vi "Manual worksheet input.vi"() -> (0 "error out":errorcluster, 1 "data names":string[](array[string]), 2 "file numbers":string[](array[string]), 3 "Data clusters":cluster{"array type (2D Dbl)":dbl[][]}[](array[cluster]))   [LabVIEW 2019]
panel:
  in  "dataset name (option)":string="data"
  in  "OK":bool=TRUE
  out "XY Graph":T1(graph)
  in  "XY data worksheet":string
  # "Worksheet has a format below (2n colums)\nx1, y1, x2, y2, x3, y3,... xn, yn\n\nConvert to datasets of individual n XY plots such as  (x1, y1), (x2, y2), ...(xn,yn)."
  # "(Copy and Paste multiple XY data set)"
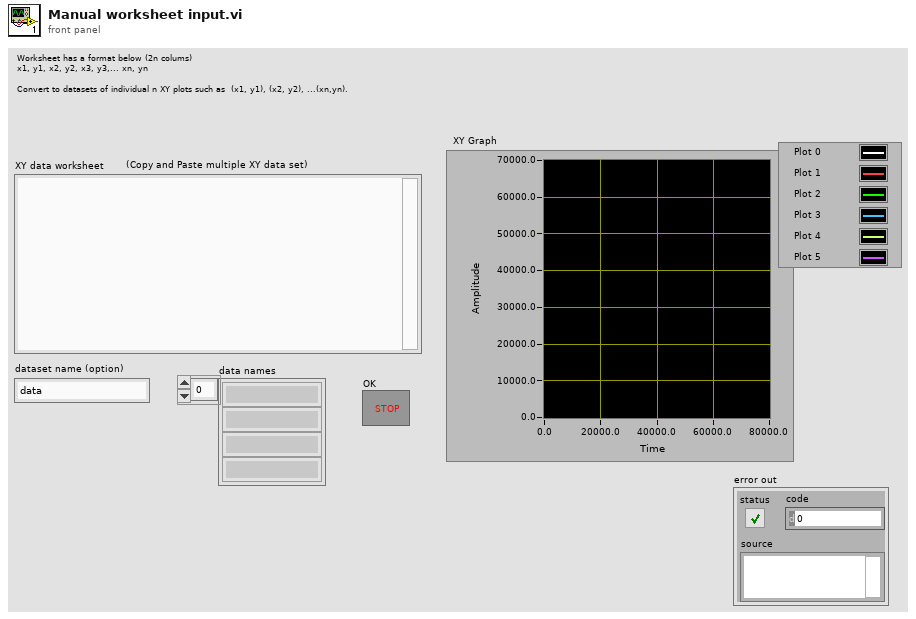
[diagram p1: front panel]
types:
  T1 = cluster{"array type (2D Dbl)":dbl[], "array type (2D Dbl)":dbl[]}[]
  T2 = cluster{"array type (2D Dbl)":dbl[], "array type (2D Dbl)":dbl[]}
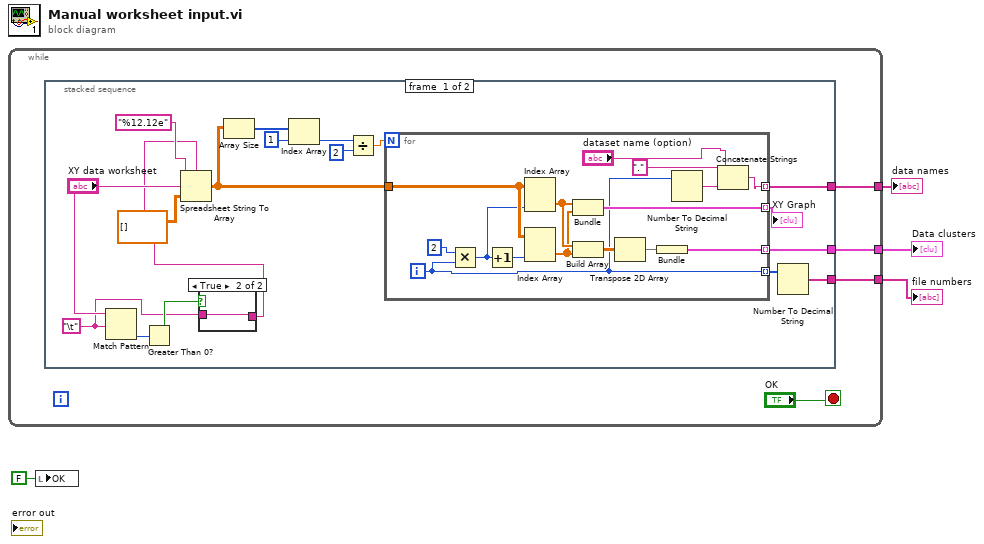
[diagram p0: block diagram]
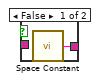
[diagram p2: hidden frame]
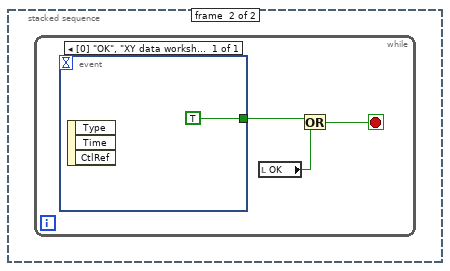
[diagram p3: hidden frame]
diagram:
  n1 = while {
    tunnel: [w8] -> w4
    tunnel: [w6] -> w3
    tunnel: [w5] -> w1
    stop <- "OK" stop-if-true
    n2 = stacked-sequence {
      tunnel: [w17 _] -> w8
      tunnel: [w15 _] -> w6
      tunnel: [w9 _] -> w5
      frame #0 {
        w11 = "\t"
        n3 = Match Pattern(string="XY data worksheet", regular expression=w11) -> (offset past match=w14:i32)  [unwired: 1 in, 3 out]
        n4 = Greater Than 0?(x=w14) -> (x > 0?=w12:bool)
        n5 = case shown="True" w12 {
          tunnel: [w27 w28] -> w10
          tunnel: w11 -> [_ w28]
          frame False {
            n6 = call <vilib>:"Space Constant.vi"() -> ("String"=w27:string)
          }
          frame True {
          }
        }
        n7 = Spreadsheet String To Array(delimiter (Tab)=w10, format string="%12.12e", spreadsheet string="XY data worksheet", array type (2D Dbl)=dbl[][] []) -> (array=w19:dbl[][])
        n8 = Array Size(array=w19) -> (size(s)=w24:i32[])
        n9 = Index Array(array=w24, index=1) -> (element=w22:i32)
        n10 = Divide(x=w22, y=2) -> (x/y=w20:dbl)
        n11 = for {
          N: w20 -> [_]
          tunnel: w19 -> [w43]
          tunnel: [w39] -> w18 mode=indexing
          tunnel: [w36] -> w17 mode=indexing
          tunnel: [w33] -> w16 mode=indexing
          tunnel: [w29] -> w9 mode=indexing
          i -> [w33]
          n12 = Multiply(x=2, y=w33) -> (x*y=w41:i32)
          n13 = Increment(x=w41) -> (x+1=w40:i32)
          n14 = Index Array(array=w43, index (col)=w41) -> (element=w38:dbl[])  [unwired: 1 in]
          n15 = Index Array(array=w43, index (col)=w40) -> (element=w37:dbl[])  [unwired: 1 in]
          n16 = Bundle("array type (2D Dbl)"=w38, "array type (2D Dbl)"=w37) -> (w39:T2)  [unwired: 1 in]
          n17 = Build Array(w38, w37) -> (w34:dbl[][])
          n18 = Transpose 2D Array(2D array=w34) -> (transposed array=w35:dbl[][])
          n19 = Bundle(w35) -> (w36:cluster{dbl[][]})  [unwired: 1 in]
          n20 = Number To Decimal String(number=w33) -> (decimal integer string=w31:string)  [unwired: 1 in]
          n21 = Concatenate Strings("dataset name (option)", "." ("string"), w31) -> (w29:string)
        }
        "XY Graph" <- w18
        n22 = Number To Decimal String(number=w16) -> (decimal integer string=w15:string[])  [unwired: 1 in]
      }
      frame #1 {
        n23 = while {
          stop <- w45 stop-if-true
          n24 = event shown="[0] \"OK\", \"XY data worksheet\": Value Change;  \"OK\": Mouse Enter;  \"OK\": Mouse Leave" {
            selector: _ -> [_]
            dyn-events: _ -> [_]
            timeout: _ -> [_]
            tunnel: [TRUE ("stop")] -> w46
            event "OK", "XY data worksheet": Value Change; "OK": Mouse Enter; "OK": Mouse Leave {
              n25 = event-data() -> ()  [unwired: 1 in, 3 out]
            }
          }
          n26 = local read "OK"() -> (w44:bool)
          n27 = Or(x=w46, y=w44) -> (x .or. y?=w45:bool)
        }
      }
    }
  }
  "file numbers" <- w3
  "Data clusters" <- w4
  "data names" <- w1
  n28 = local write "OK"(FALSE ("OK")) -> ()
